vi "Airheater model and real.vi"() -> ()   [LabVIEW 2019]
uses:
  <vilib>/Simulation/Scripting/Companion Diagram/SimConfigNode/SimParams.ctl
  <vilib>/Simulation/Scripting/Companion Diagram/SimConfigNode/_simSolvers.ctl
  <vilib>/Simulation/Implementation/Shared/SIMSCR Execution Mode.ctl
  <vilib>/Simulation/Param Hierarchy/Typedefs/SIMPH Param Control Actions.ctl
  <vilib>/Simulation/Implementation/Shared/NILVSim_ParamChanged.vi
  <vilib>/Simulation/Implementation/Shared/NILVSIM_BeginStep.vi
  <vilib>/Simulation/Implementation/Shared/NILVSim_Manager.vi
  <vilib>/Utility/error.llb/Clear Errors.vi
  <vilib>/Simulation/Implementation/Shared/NILVSim_FinalizeModel.vi
  <vilib>/DAQmx/read.llb/DAQmx Read (Analog DBL 1Chan 1Samp).vi
  <vilib>/DAQmx/write.llb/DAQmx Write (Analog DBL 1Chan 1Samp).vi
  <vilib>/Simulation/Implementation/Shared/SIM Unbundle Sim Info.vi
  <vilib>/Simulation/Implementation/Shared/NILVSim_Initialize.vi
  <vilib>/Simulation/Utility/Implementation/NILVSim Get Time and IsAcceptedStep.vi
  <vilib>/Simulation/Implementation/Shared/SIMSH Read Queue.vi
  <vilib>/Simulation/Implementation/Shared/NILVSim_GetModelError.vi
  <vilib>/Simulation/Implementation/Shared/SIM Bundle Sim Info.vi
  <vilib>/DAQmx/miscellaneous.llb/DAQmx Fill In Error Info.vi
  <vilib>/Simulation/Implementation/XNodeFramework/SimXNode/SimX.xnode
  Airheater Model subsystem.vi
  <vilib>/Simulation/Scripting/Companion Diagram/SimConfigNode/SimDog.xnode
  Air Heater Black Box Model.vi
  <vilib>/Simulation/Implementation/Shared/NI_SIM_Implementation.lvlib
panel:
  in  "Set point":dbl(slide)=20.0 min=20.0 max=50.0 scale=20.0..50.0
  in  "Ti":dbl
  in  "Kp":dbl
  in  "Real":bool
  out "Control Signal Chart":dbl(graph)
  out "Temperature Chart":T1(graph)
  in  "stop":bool
  in  "Delay [s]":dbl=2.9
  in  "Time constant [s]":dbl=15.0
  in  "T_enviroment [C]":dbl=24.3
  in  "K [C/V]":dbl=2.1
  out "Task AO":refnum<k21>
  out "Task AI":refnum<k21>
  # "PI Controller parameters"
  # "Model parameters"
  # "Blackbox"
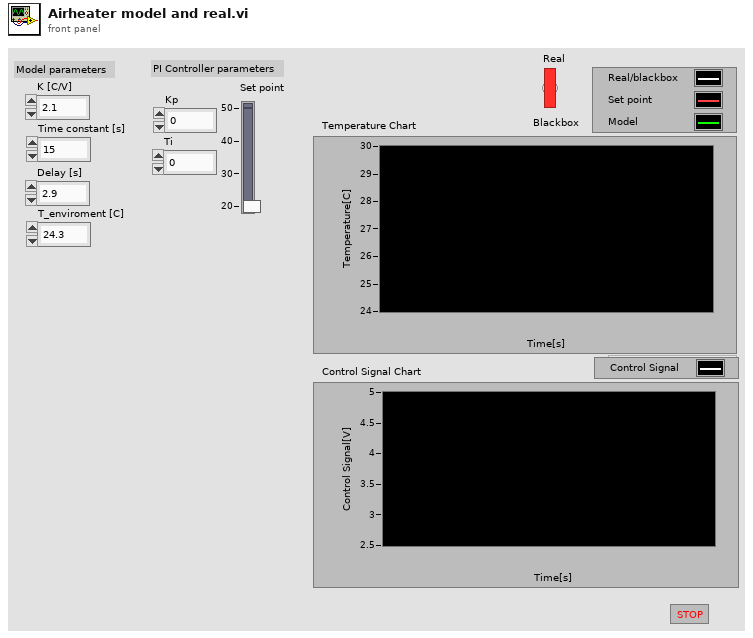
[diagram p1: front panel]
types:
  T1 = cluster{"Filter Output":dbl, "Set point":dbl, "T_out [C]":dbl}
  T2 = cluster{"Filter Output":dbl, "Set point":dbl, "T_out [C]":dbl}[]
  T3 = enum16{"Simulate to Completion", "Single Time-Step Simulation (Fixed Step Only)"}
  T4 = typedef "SIMSCR Execution Mode.ctl" = enum16{"Simulate to Completion", "Single Time-Step Simulation (Fixed Step Only)"}
  T5 = typedef "SIMPH Param Control Actions.ctl" = enum16{"get params", "set params"}
  T6 = cluster{"SIMSH Sim Time":dbl, "Select":cluster{"s? t:f":dbl}, "Linear Scaling with Points.vi":cluster{"y":dbl}, "Summation 3":cluster{"Result":dbl}, "Square Root":cluster{"sqrt(x)":dbl}, "Gaussian White Noise PtByPt.vi":cluster{"Gaussian white noise":dbl}, "Integrator":cluster{"output":dbl}, "Multiplication":cluster{"Result":dbl}, "Summation":cluster{"Result":dbl}, "Multiplication 2":cluster{"Result":dbl}, "Transport Delay":cluster{"output":dbl}, "Summation 2":cluster{"Result":dbl}}
  T7 = typedef "SimParams.ctl" = cluster{"Initial Time (s)":dbl, "Final Time (s)":dbl, "Step Size (s)":dbl, "ODE Solver":T8, "Minimum Step Size (s)":dbl, "Maximum Step Size (s)":dbl, "Relative Tolerance":dbl, "Absolute Tolerance":dbl, "Software Timing":bool, "Initial Step Size (s)":dbl, "Automatic Fixed Step Size?":bool, "Automatic Discrete Step Size?":bool, "Discrete Step Size (s)":dbl, "Calculate using Time Step":bool, "Solver Wired?":bool, "Prev.Frm.Expected End":u64, "Prev.Frm.Actual End":u64, "Prev.Frm.Finished Late?":bool, "Prev.Iter.Expected End":u64, "Prev.Iter.Actual End":u64, "Prev.Iter.Finished Late?":bool, "Expected Iteration Start":u64, "Actual Iteration Start":u64, "Expected Frame Start":u64, "Actual Frame Start":u64, "Source Name":string, "Name":string, "Period":i64, "Deadline":i64, "Offset":i64, "Start":i64, "Priority":i32, "Timeout":i32, "Processor":i32, "Mode":enum32{"No Change", "Process missed periods, maintain original phase", "Discard missed periods, maintain original phase", "Process missed periods, ignore original phase", "Discard missed periods, ignore original phase"}, "Wakeup reason":enum32{"Normal", "Aborted", "Asynchronous wakeup", "Timing source error", "Timed loop error", "Timeout"}, "Error":errorcluster, "Source Type":string, "Secondary Source Type":string, "Global End Time":u64, "Global Start Time":u64, "Full Solver Reset":bool, "Execution Mode":T4, "Nan/Inf Check":bool, "Custom Solver Library":string, "Solver Is Variable":bool, "custom solver name":string, "Signal Collection Decimation":u32}
  T8 = typedef "_simSolvers.ctl" = enum16{"Runge-Kutta 1 (Euler)", "Runge-Kutta 2", "Runge-Kutta 3", "Runge-Kutta 4", "Runge-Kutta 23 (variable)", "Runge-Kutta 45 (variable)", "BDF (variable)", "Adams-Moulton (variable)", "Rosenbrock (variable)", "Discrete States Only", "SDIRK 4 (variable)", "Radau 5 (variable)", "Radau 9 (variable)", "Radau 13 (variable)", "Radau [Variable Order] (variable)", "Gear's Method (variable)", "Linearizer", "State Query", "Trim Eval", "Custom Solver"}
  T9 = cluster{"SIMSH Sim Time":dbl, "Operand2":dbl, "Multiplication 3":cluster{"Result":dbl}, "Integrator":cluster{"output":dbl}, "Multiplication 2":cluster{"Result":dbl}, "Summation 2":cluster{"Result":dbl}, "Transport Delay":cluster{"output":dbl}, "Summation":cluster{"Result":dbl}, "Multiplication":cluster{"Result":dbl}}
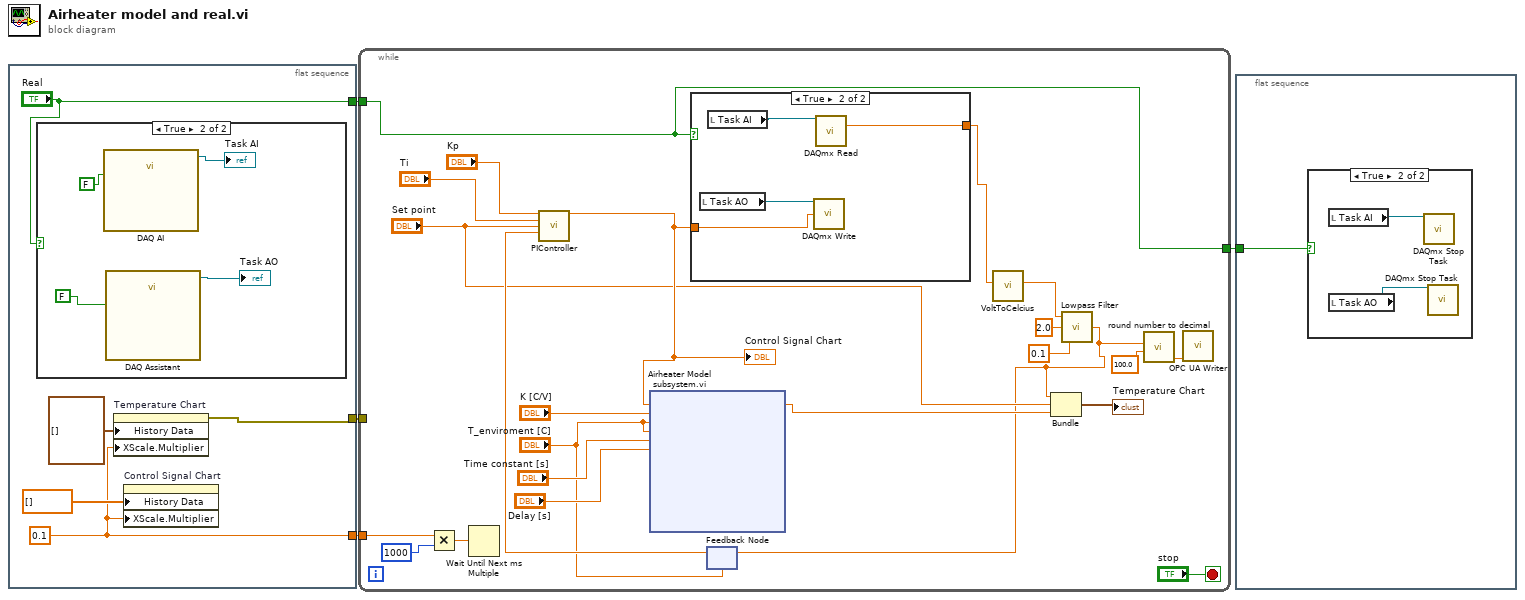
[diagram p0: block diagram]
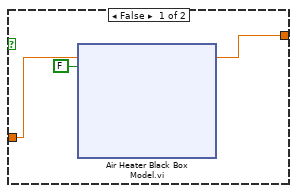
[diagram p4: hidden frame]
diagram:
  n1 = flat-sequence {
    tunnel: [w9] -> w4
    tunnel: [w7] -> w3
    tunnel: ["Real"] -> w2
    frame #0 {
      w7 = 0.1
      n2 = case shown="True" "Real" {
        frame False {
        }
        frame True {
          n3 = call "DAQ AI"("stop (T)"=FALSE) -> ("task out"=→"Task AI":refnum<k21>)  [unwired: 16 in, 2 out]
          n4 = call "DAQ Assistant"("stop (T)"=FALSE) -> ("task out"=→"Task AO":refnum<k21>)  [unwired: 17 in, 1 out]
        }
      }
      n5 = property on="Temperature Chart" class="WFChart (strict)"("History Data"=T2 [], "XScale.Multiplier"=w7) -> (error out=w9:errorcluster)  [unwired: 2 in, 1 out]
      n6 = property on="Control Signal Chart" class="WFChart (strict)"("History Data"=dbl[] [], "XScale.Multiplier"=w7) -> ()  [unwired: 2 in, 2 out]
    }
  }
  n7 = while {
    tunnel: w4 -> [_]
    tunnel: w3 -> [w30]
    tunnel: w2 -> [w25]
    tunnel: [w25] -> w1
    stop <- "stop" stop-if-true
    n8 = Multiply(x=w30, y=u32 1000 ("millisecond multiple")) -> (x*y=w32:dbl)
    n9 = Wait Until Next ms Multiple(millisecond multiple=w32) -> ()  [unwired: 1 out]
    n10 = feedback #1("T_enviroment [C]") -> (w20:dbl)
    n11 = call "PIController.vi"("Kp"="Kp", "Ti"="Ti", "setP"="Set point", "temp"=w20) -> ("Control Signal"=w23:dbl)  [unwired: 11 in]
    "Control Signal Chart" <- w23
    n12 = xnode "Airheater Model subsystem.vi"("u [V]"=w23, "K [C/V]"="K [C/V]", "T_enviroment [C]"="T_enviroment [C]", "T_initial [C]"="T_enviroment [C]", "Time constant [s]"="Time constant [s]", "Delay [s]"="Delay [s]") -> ("T_out [C]"=w15:dbl)  [unwired: 2 in, 14 out]
    n13 = case shown="True" w25 {
      tunnel: w23 -> [w39 w288]
      tunnel: [w38 w287] -> w24
      frame False {
        n14 = xnode "Air Heater Black Box Model.vi"("Control Signal [0-5V]"=w39, "Initialize"=FALSE) -> ("Tout [1-5V]"=w38:dbl)  [unwired: 1 in, 1 out]
      }
      frame True {
        n15 = local read "Task AO"() -> (w285:refnum<k21>)
        n16 = local read "Task AI"() -> (w286:refnum<k21>)
        n17 = call-poly <vilib>:"DAQmx Write.vi"("task/channels in"=w285, "data"=w288) -> ()  [unwired: 11 in, 3 out]
        n18 = call-poly <vilib>:"DAQmx Read.vi"("task/channels in"=w286) -> ("data"=w287:dbl)  [unwired: 12 in, 2 out]
      }
    }
    n19 = call "VoltToCelcius.vi"("Voltage"=w24) -> ("Temperature[C]"=w26:dbl)  [unwired: 10 in]
    n20 = call "Lowpass Filter.vi"("Ts [s]"=0.1, "Tf [s]"=2.0, "Filter Input"=w26) -> ("Filter Output"=w14:dbl)
    n21 = feedback-in #1(w14) -> ()
    n22 = Bundle("Filter Output"=w14, "Set point"="Set point", "T_out [C]"=w15) -> (→"Temperature Chart":T1)  [unwired: 1 in]
    n23 = call "round number to decimal.vi"("y"=100.0, "x"=w14) -> ("rounded number"=w18:dbl)  [unwired: 9 in]
    n24 = call "OPC UA Writer.vi"("Temperature"=w18) -> ()  [unwired: 11 in]
  }
  n25 = flat-sequence {
    tunnel: w1 -> [w561]
    frame #0 {
      n26 = case shown="True" w561 {
        frame False {
        }
        frame True {
          n27 = local read "Task AI"() -> (w562:refnum<k21>)
          n28 = local read "Task AO"() -> (w563:refnum<k21>)
          n29 = call <vilib>:"DAQmx Stop Task.vi"("task/channels in"=w562) -> ()  [unwired: 13 in, 2 out]
          n30 = call <vilib>:"DAQmx Stop Task.vi"("task/channels in"=w563) -> ()  [unwired: 13 in, 2 out]
        }
      }
    }
  }
